vi "getSheetDim.vi"(8 "error in (no error)":errorcluster, 9 "sheetName":string, 10 "filePath":string, 11 "reference in":refnum<class "python.lvclass">) -> (0 "error out":errorcluster, 2 "sheetsDim(Row,Column)":string[](array[string]), 3 "reference out":refnum<class "python.lvclass">)   [LabVIEW 2014, in "python.lvclass"]
uses:
  python.lvclass
  <vilib>/Utility/error.llb/DialogType.ctl
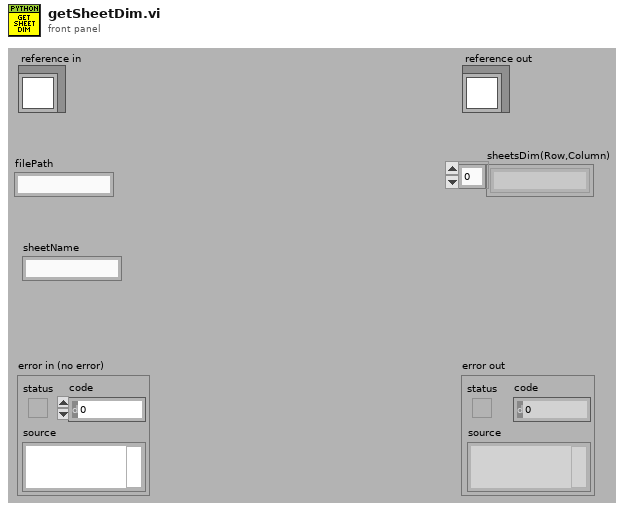
[diagram p1: front panel]
types:
  T1 = typedef "python.lvclass/ObjectAttributesRef.ctl" = refnum<data-value>
  T2 = typedef "python.lvclass/ObjectAttributes.ctl" = cluster{"MyAttribute":dbl, "workingDirectory":path}
  T3 = typedef "DialogType.ctl" = u16
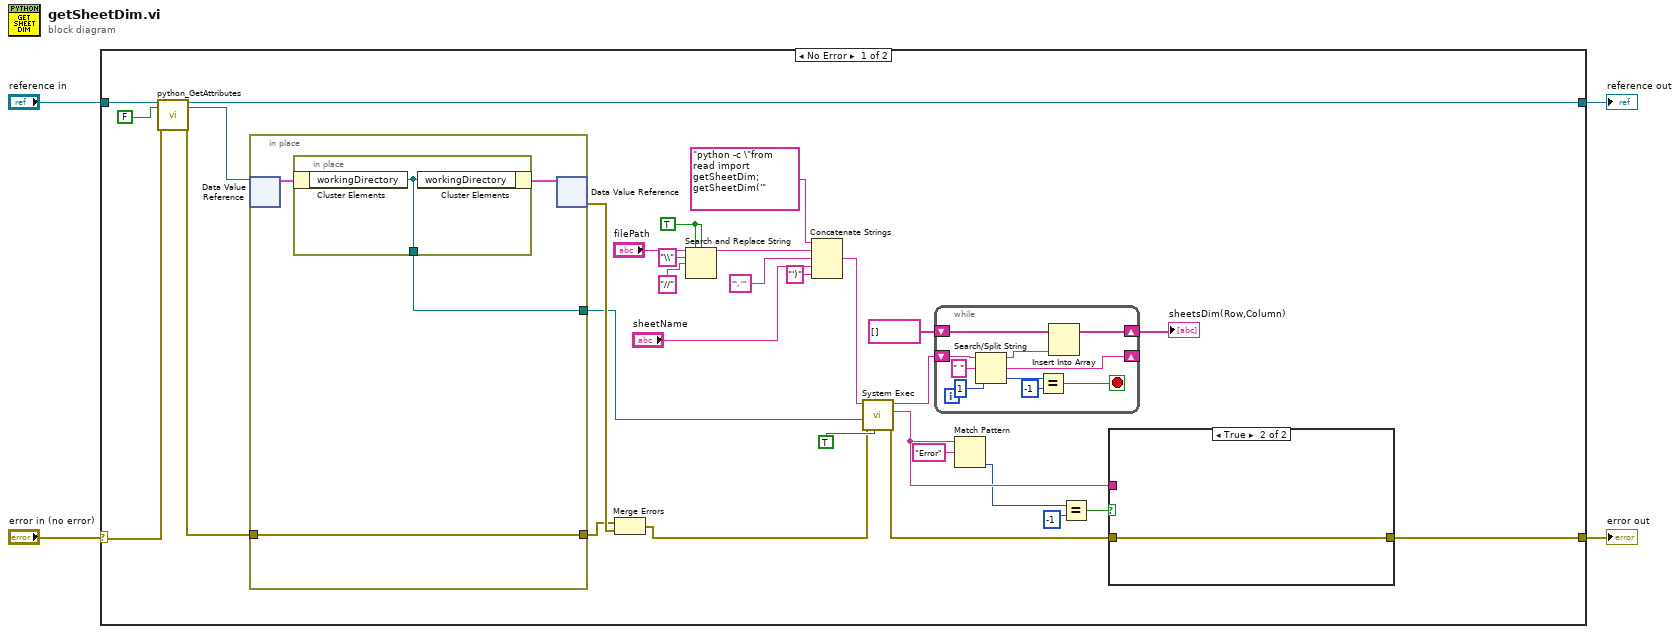
[diagram p0: block diagram]
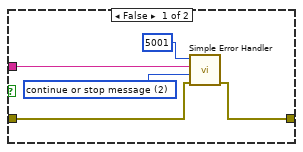
[diagram p2: hidden frame]
diagram:
  n1 = case shown="No Error" "error in (no error)" {
    selector: "error in (no error)" -> [w31 w58]
    tunnel: [w18 w58] -> w3
    tunnel: [w29 w57] -> w1
    tunnel: "reference in" -> [w33 w57]
    frame No Error {
      w13 = TRUE ("replace all? (F)")
      n2 = call "python_GetAttributes.vi"("reference in"=w33, "return data? (T)"=FALSE, "error in (no error)"=w31) -> ("reference out"=w29:refnum<class "python.lvclass">, "attributes ref"=w28:T1, "error out"=w30:errorcluster)  [unwired: 13 in, 1 out]
      n3 = in-place {
        in-place-border: w30 -> [w53]
        in-place-border: [w53] -> w34
        in-place-border: [w52] -> w26
        n4 = in-place-dvr #1(w28) -> (w54:T2)  [unwired: 1 out]
        n5 = in-place {
          in-place-border: [w56] -> w52
          n6 = in-place-cluster #2(w54) -> ("workingDirectory"=w56:path)
          n7 = in-place-cluster #2("workingDirectory"=w56) -> (w55:T2)
        }
        n8 = in-place-dvr #1(w55) -> (w35:errorcluster)  [unwired: 1 out]
      }
      n9 = Merge Errors(w34, w35) -> (w25:errorcluster)
      n10 = Search and Replace String(replace all?=w13, case sensitive?=w13, input string="filePath", search string="\\", replace string="//" ("search string")) -> (result string=w14:string)  [unwired: 3 in, 3 out]
      n11 = Concatenate Strings("python -c \"from read import getSheetDim; getSheetDim('" ("string"), w14, "', '" ("string"), "sheetName", "')" ("string")) -> (w22:string)
      n12 = call <vilib>:"System Exec.vi"("run minimized? (F)"=TRUE, "error in (no error)"=w25, "working directory"=w26, "command line"=w22) -> ("error out"=w19:errorcluster, "standard error"=w12:string, "standard output"=w20:string)  [unwired: 2 in, 3 out]
      n13 = while {
        shift-right: [w50] -> w5
        shift-left: string[] [] -> [w51]
        shift-right: [w46] -> _
        shift-left: w20 -> [w49]
        stop <- w44 stop-if-true
        n14 = Search/Split String(string=w49, search string/char (-)=" ", offset (0)=1) -> (substring before match=w48:string, match + rest of string=w46:string, offset of match=w45:i32)
        n15 = Equal?(x=w45, y=-1) -> (x = y?=w44:bool)
        n16 = Insert Into Array(array=w51, new element=w48) -> (w50:string[])  [unwired: 1 in]
      }
      "sheetsDim(Row,Column)" <- w5
      n17 = Match Pattern(string=w12, regular expression="Error") -> (offset past match=w8:i32)  [unwired: 1 in, 3 out]
      n18 = Equal?(x=w8, y=-1 ("offset past match")) -> (x = y?=w9:bool)
      n19 = case shown="True" w9 {
        tunnel: w19 -> [w40 w41]
        tunnel: [w39 w41] -> w18
        tunnel: w12 -> [w37 _]
        frame False {
          w36 = T3 2 items=["no dialog", "OK message", "continue or stop message", "OK message + warnings", "continue/stop + warnings"] ("type of dialog (OK msg:1)")
          n20 = call <vilib>:"Simple Error Handler.vi"("error code (no error:0)"=5001, "error source (\" \")"=w37, "type of dialog (OK msg:1)"=w36, "error in (no error)"=w40) -> ("error out"=w39:errorcluster)  [unwired: 5 out]
        }
        frame True {
        }
      }
    }
    frame Error {
    }
  }
  "error out" <- w3
  "reference out" <- w1
